vi "Dpc Query Config Status.vi"(7 "perc":i32, 8 "error in (no error)":errorcluster, 9 "ptrs":T1, 10 "trid":u16, 11 "hif":u32) -> (0 "error out":errorcluster, 1 "ptrs out":T1, 2 "function return":i32, 3 "hif out":u32, 5 "perc out":i32)   [LabVIEW 2011, in "LVH-Adept.lvlib" / "DPCUTIL.lvlib"]
doc: "DPCAPI BOOL DpcQueryConfigStatus(HANDLE hif, TRID trid, TRS * ptrs, ERC * perc);"
uses:
  DPCUTIL.lvlib
  Resources/dpcutil.dll
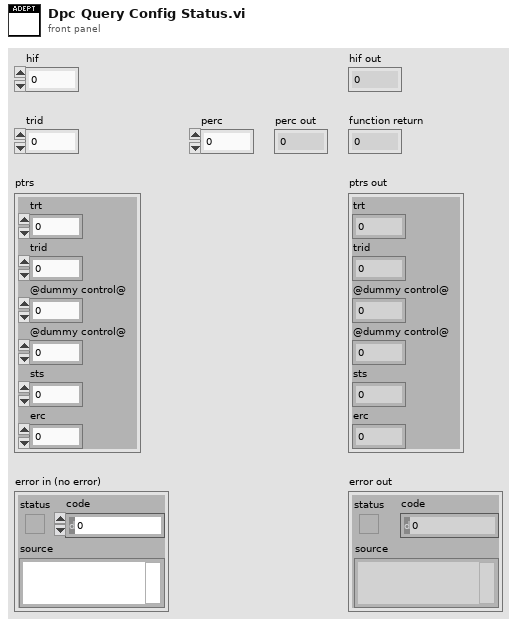
[diagram p1: front panel]
types:
  T1 = cluster{"trt":i32, "trid":u16, "@dummy control@":i8, "@dummy control@":i8, "sts":i32, "erc":i32}
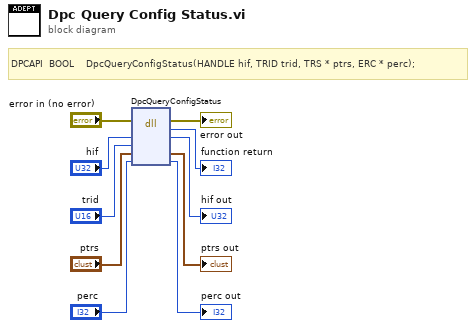
[diagram p0: block diagram]
diagram:
  # "DPCAPI  BOOL    DpcQueryConfigStatus(HANDLE hif, TRID trid, TRS * ptrs, ERC * perc);"
  n1 = dll-call lib="C:/github/labviewhacker/LVH-Adept/LabVIEW/vi.lib/LabVIEW Hacker/Adept/Private/Resources/dpcutil.*" fn="DpcQueryConfigStatus"(error in="error in (no error)", "hif"="hif", "trid"="trid", "ptrs"="ptrs", "perc"="perc") -> (error out=→"error out":errorcluster, →"function return":i32, "hif"=→"hif out":u32, "ptrs"=→"ptrs out":T1, "perc"=→"perc out":i32)  [unwired: 3 in, 1 out]
